vi "addLayout.vi"(8 "Error In":errorcluster, 9 "stretch":i32, 10 "layout":refnum<class "QLayout.lvclass">, 11 "QBoxLayout In":refnum<class "QBoxLayout.lvclass">) -> (0 "Error Out":errorcluster, 3 "QBoxLayout Out":refnum<class "QBoxLayout.lvclass">)   [LabVIEW 2014, in "QBoxLayout.lvclass"]
doc: "LabVIEW-specific documentation is not yet available. See <b>http://doc.qt.io/qt-5/QBoxLayout.html#addLayout</b>"
uses:
  QBoxLayout.lvclass
  QLayout/QLayout.lvclass
  LQ Core/LQIdentity/LQIdentity.lvclass/LQIdentity.ctl
  LQ Core/LQ Core.lvlib
  LQ Core/LQIdentity/LQIdentity.lvclass
panel:
  # "Copyright (c) 2016 Sze Howe Koh\n\nThis Source Code Form is subject to the terms of the Mozilla Public\nLicense, v. 2.0. If a copy of the MPL was not distributed with this\nfile, You can obtain one at http://mozilla.org/MPL/2.0/."
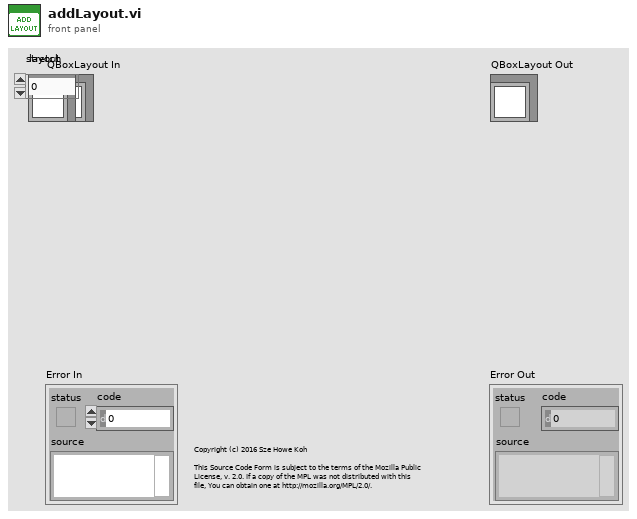
[diagram p1: front panel]
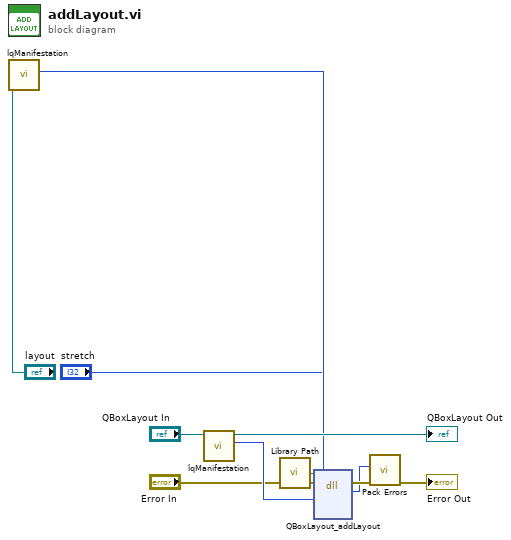
[diagram p0: block diagram]
diagram:
  n1 = call "lqManifestation.vi"("LQIdentity in"="layout") -> ("Manifestation"=w2:u64)  [unwired: 9 in, 1 out]
  n2 = call "lqManifestation.vi"("LQIdentity in"="QBoxLayout In") -> ("Manifestation"=w8:u64, "LQIdentity out"=→"QBoxLayout Out":refnum<class "QBoxLayout.lvclass">)  [unwired: 9 in]
  n3 = call "Library Path.vi"() -> ("Library Path"=w9:path)
  n4 = dll-call lib="?" fn="QBoxLayout_addLayout"(path in=w9, error in="Error In", "_instance"=w8, "layout"=w2, "stretch"="stretch") -> (error out=w6:errorcluster, w4:i32)  [unwired: 4 in, 1 out]
  n5 = call "Pack Errors.vi"("Error In"=w6, "Error Code"=w4) -> ("Error Out"=→"Error Out":errorcluster)  [unwired: 9 in]
